vi "INIT shooter.vi"(8 "error in (no error)":errorcluster) -> (0 "error out":errorcluster)   [LabVIEW 2023]
uses:
  <vilib>/Rock Robotics/WPI/ThirdParty/REV Robotics/REVLib/Typedef/Spark MAX Sensor Type.ctl
  Global INIT.vi
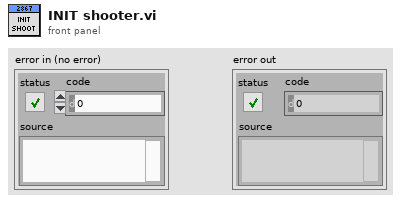
[diagram p1: front panel]
types:
  T1 = typedef "Spark MAX Sensor Type.ctl" = enum16{"No Sensor", "Hall Sensor", "Encoder", "-Not Available-", "Analog", "Alternate Encoder", "Duty Cycle"}
  T2 = typedef "ctrl swerve motor.ctl" = cluster{"description":string, "Installed?":bool, "CAN ID":u8, "refnum name":string, "Invert":bool, "Idle Mode":T3, "Current limiting":T4}
  T3 = typedef "Spark MAX Idle Mode.ctl" = enum16{"Coast", "Brake"}
  T4 = typedef "ctrl Spark MAX current limiting.ctl" = cluster{"Linearized Limit Enabled (F)":bool, "Free Speed Current Limit (20A)":dbl, "Primay Current Limit (80A)":dbl, "Linear Limit RPM (0)":u32}
  T5 = typedef "WPI_MotorControlDeviceRef.ctl" = cluster{"DeviceStatus":errorcluster, "Type":T6, "PWM":cluster{"PWM Channel":T7, "DeadBand":T8}, "CAN":cluster{"Device Number":u8, "SetOutput VI Ref":variant, "GetOutput VI Ref":variant, "Enable VI Ref":variant, "Disable VI Ref":variant, "Data":variant}, "Invert":bool, "DIO PWM":cluster{"PWM \"Enable\" Channel":T7, "DIOChannel":T9, "PWM Rate":dbl}}
  T6 = typedef "WPI_MotorControlType.ctl" = enum16{"PWM", "CAN", "DIO PWM"}
  T7 = typedef "FPGA_DIOPWMChannel.ctl" = enum8{"PWM 0", "PWM 1", "PWM 2", "PWM 3", "PWM 4", "PWM 5", "PWM 6", "PWM 7", "PWM 8", "PWM 9", "PWM MXP 0", "PWM MXP 1", "PWM MXP 2", "PWM MXP 3", "PWM MXP 4", "PWM MXP 5", "PWM MXP 6", "PWM MXP 7", "PWM MXP 8", "PWM MXP 9", "Invalid"}
  T8 = typedef "WPI_PWMDeadband.ctl" = cluster{"Name":string, "maxPositivePwm":i32, "minPositivePwm":i32, "centerPwm":i32, "maxNegativePwm":i32, "minNegativePwm":i32, "angularRange":u16}
  T9 = typedef "FPGA_DIOChannel.ctl" = enum8{"DIO 0", "DIO 1", "DIO 2", "DIO 3", "DIO 4", "DIO 5", "DIO 6", "DIO 7", "DIO 8", "DIO 9", "DIO MXP 0", "DIO MXP 1", "DIO MXP 2", "DIO MXP 3", "DIO MXP 4", "DIO MXP 5", "DIO MXP 6", "DIO MXP 7", "DIO MXP 8", "DIO MXP 9", "DIO MXP 10", "DIO MXP 11", "DIO MXP 12", "DIO MXP 13", "DIO MXP 14", "DIO MXP 15", "SPI Port CS1", "SPI Port CS2", "SPI Port CS3", "SPI Port MISO", "SPI Port MOSI", "Invalid"}
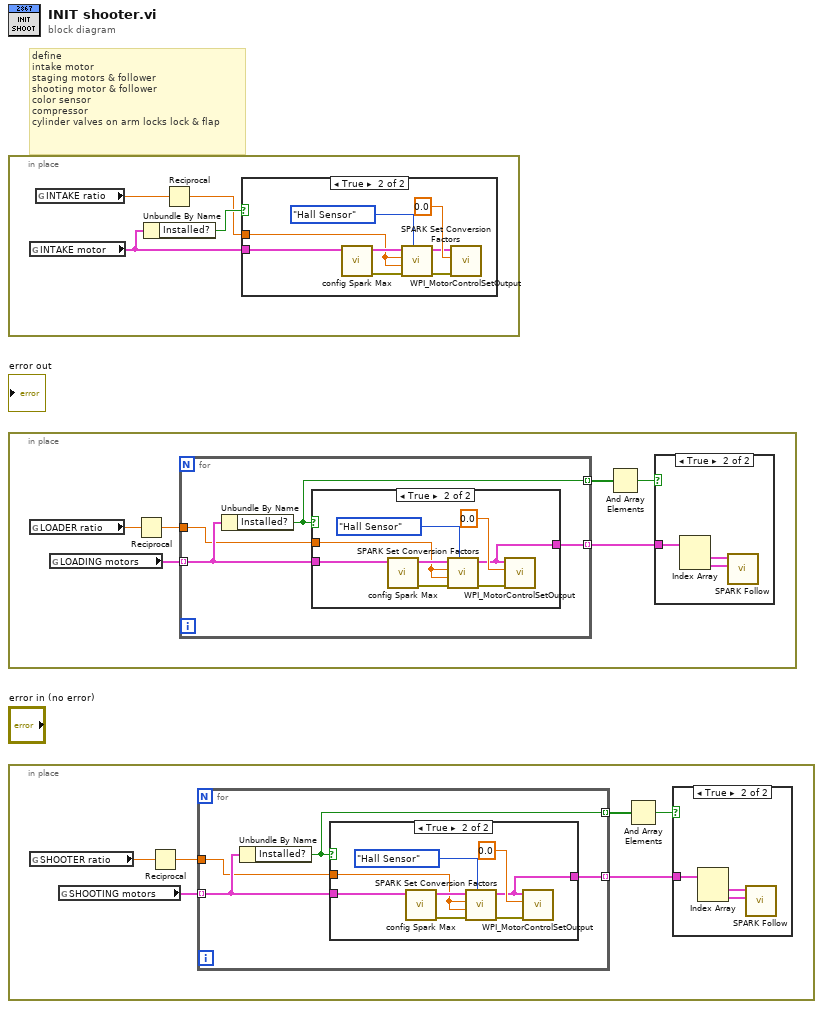
[diagram p0: block diagram]
diagram:
  # "define\nintake motor\nstaging motors & follower\nshooting motor & follower\ncolor sensor\ncompressor\ncylinder valves on arm locks lock & flap"
  n1 = in-place {
    n2 = global read "Global INIT.vi" "INTAKE motor"() -> (w3:T2)
    n3 = global read "Global INIT.vi" "INTAKE ratio"() -> (w2:dbl)
    n4 = Unbundle By Name(w3) -> ("Installed?"=w4:bool)
    n5 = Reciprocal(x=w2) -> (1/x=w1:dbl)
    n6 = case shown="True" w4 {
      tunnel: w3 -> [_ w10]
      tunnel: w1 -> [_ w5]
      frame False {
      }
      frame True {
        n7 = call "config Spark Max.vi"("motor\ndefaults"=w10) -> ("error out"=w6:errorcluster, "MotorControlDevRef"=w7:T5)  [unwired: 9 in]
        n8 = call <vilib>:"SPARK Set Conversion Factors.vi"("Sensor Type (Hall Sensor)"=Spark_MAX_Sensor_Type."Hall Sensor", "error in (no error)"=w6, "Velocity Factor (1)"=w5, "Position Factor (1)"=w5, "MotorControlDeviceRef in"=w7) -> ("error out"=w8:errorcluster, "MotorControlDeviceRef out"=w9:T5)  [unwired: 5 in]
        n9 = call <vilib>:"WPI_MotorControlSetOutput.vi"("error in (no error)"=w8, "Output"=0.0, "MotorControlDevRef"=w9) -> ()  [unwired: 6 in, 3 out]
      }
    }
  }
  n10 = in-place {
    n11 = global read "Global INIT.vi" "LOADER ratio"() -> (w14:dbl)
    n12 = global read "Global INIT.vi" "LOADING motors"() -> (w18:T2[])
    n13 = Reciprocal(x=w14) -> (1/x=w13:dbl)
    n14 = for {
      tunnel: w18 -> [w25] mode=indexing
      tunnel: [w24] -> w17 mode=indexing
      tunnel: [w23] -> w16 mode=indexing
      tunnel: w13 -> [w22]
      n15 = Unbundle By Name(w25) -> ("Installed?"=w23:bool)
      n16 = case shown="True" w23 {
        tunnel: w25 -> [_ w30]
        tunnel: [_ w27] -> w24
        tunnel: w22 -> [_ w26]
        frame False {
        }
        frame True {
          n17 = call "config Spark Max.vi"("motor\ndefaults"=w30) -> ("error out"=w28:errorcluster, "MotorControlDevRef"=w29:T5)  [unwired: 9 in]
          n18 = call <vilib>:"SPARK Set Conversion Factors.vi"("Sensor Type (Hall Sensor)"=Spark_MAX_Sensor_Type."Hall Sensor", "error in (no error)"=w28, "Velocity Factor (1)"=w26, "Position Factor (1)"=w26, "MotorControlDeviceRef in"=w29) -> ("error out"=w31:errorcluster, "MotorControlDeviceRef out"=w27:T5)  [unwired: 5 in]
          n19 = call <vilib>:"WPI_MotorControlSetOutput.vi"("error in (no error)"=w31, "Output"=0.0, "MotorControlDevRef"=w27) -> ()  [unwired: 6 in, 3 out]
        }
      }
    }
    n20 = And Array Elements(Boolean array=w16) -> (logical AND=w15:bool)
    n21 = case shown="True" w15 {
      tunnel: w17 -> [_ w21]
      frame False {
      }
      frame True {
        n22 = Index Array(array=w21) -> (element #1=w20:T5, element #2=w19:T5)  [unwired: 2 in]
        n23 = call <vilib>:"SPARK Follow.vi"("Master Controller"=w19, "MotorControlDeviceRef"=w20) -> ()  [unwired: 8 in, 2 out]
      }
    }
  }
  n24 = in-place {
    n25 = global read "Global INIT.vi" "SHOOTER ratio"() -> (w36:dbl)
    n26 = global read "Global INIT.vi" "SHOOTING motors"() -> (w39:T2[])
    n27 = Reciprocal(x=w36) -> (1/x=w35:dbl)
    n28 = for {
      tunnel: w39 -> [w46] mode=indexing
      tunnel: [w45] -> w38 mode=indexing
      tunnel: [w44] -> w37 mode=indexing
      tunnel: w35 -> [w43]
      n29 = Unbundle By Name(w46) -> ("Installed?"=w44:bool)
      n30 = case shown="True" w44 {
        tunnel: w46 -> [_ w51]
        tunnel: [_ w48] -> w45
        tunnel: w43 -> [_ w47]
        frame False {
        }
        frame True {
          n31 = call "config Spark Max.vi"("motor\ndefaults"=w51) -> ("error out"=w49:errorcluster, "MotorControlDevRef"=w50:T5)  [unwired: 9 in]
          n32 = call <vilib>:"SPARK Set Conversion Factors.vi"("Sensor Type (Hall Sensor)"=Spark_MAX_Sensor_Type."Hall Sensor", "error in (no error)"=w49, "Velocity Factor (1)"=w47, "Position Factor (1)"=w47, "MotorControlDeviceRef in"=w50) -> ("error out"=w52:errorcluster, "MotorControlDeviceRef out"=w48:T5)  [unwired: 5 in]
          n33 = call <vilib>:"WPI_MotorControlSetOutput.vi"("error in (no error)"=w52, "Output"=0.0, "MotorControlDevRef"=w48) -> ()  [unwired: 6 in, 3 out]
        }
      }
    }
    n34 = And Array Elements(Boolean array=w37) -> (logical AND=w34:bool)
    n35 = case shown="True" w34 {
      tunnel: w38 -> [_ w42]
      frame False {
      }
      frame True {
        n36 = Index Array(array=w42) -> (element #1=w41:T5, element #2=w40:T5)  [unwired: 2 in]
        n37 = call <vilib>:"SPARK Follow.vi"("Master Controller"=w40, "MotorControlDeviceRef"=w41) -> ()  [unwired: 8 in, 2 out]
      }
    }
  }
